vi "svx_Map Domains for Limit Testing.vi"(0 "X signal":dbl[](array[numeric]), 1 "domain mapping":T2(ring), 5 "Y signal":dbl[](array[numeric]), 7 "X limit":dbl[](array[numeric]), 9 "Y limit":dbl[](array[numeric]), 11 "error in (no error)":errorcluster, 12 "interpolated plot mapping":T1(ring)) -> (4 "X signal out":dbl[](array[numeric]), 6 "Y signal out":dbl[](array[numeric]), 8 "X limit out":dbl[](array[numeric]), 10 "Y limit out":dbl[](array[numeric]) format="%.2f", 15 "error out":errorcluster)   [LabVIEW 2017]
uses:
  <vilib>/Analysis/1siggen.llb/Ramp Pattern by Samples.vi
  <vilib>/Analysis/NI_AALBase.lvlib
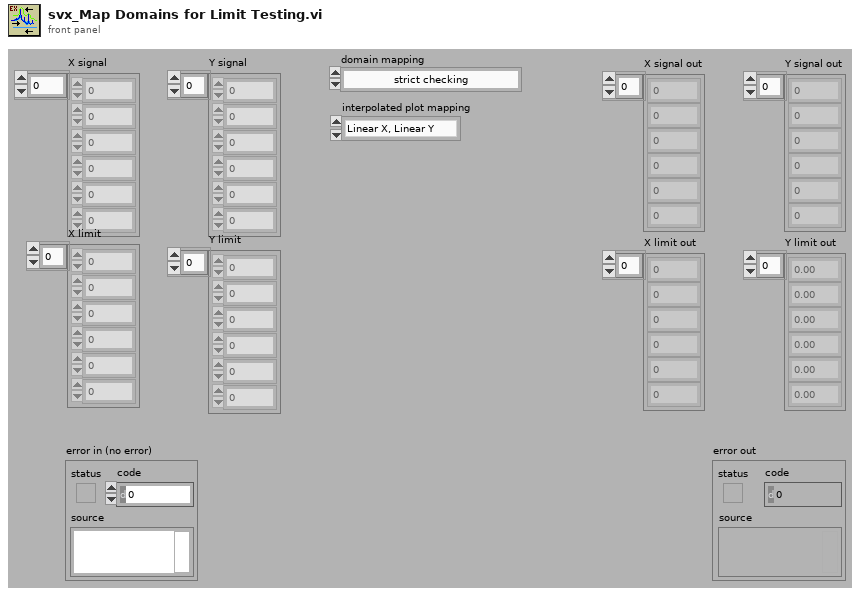
[diagram p1: front panel]
types:
  T1 = enum16{"Linear X, Linear Y", "Linear X, Log Y", "Log X, Linear Y", "Log X, Log Y"}
  T2 = enum16{"strict checking", "interpolate signal domain", "map limits to signal domain", "map signal to limit domain", "map signal and limits to unit domain"}
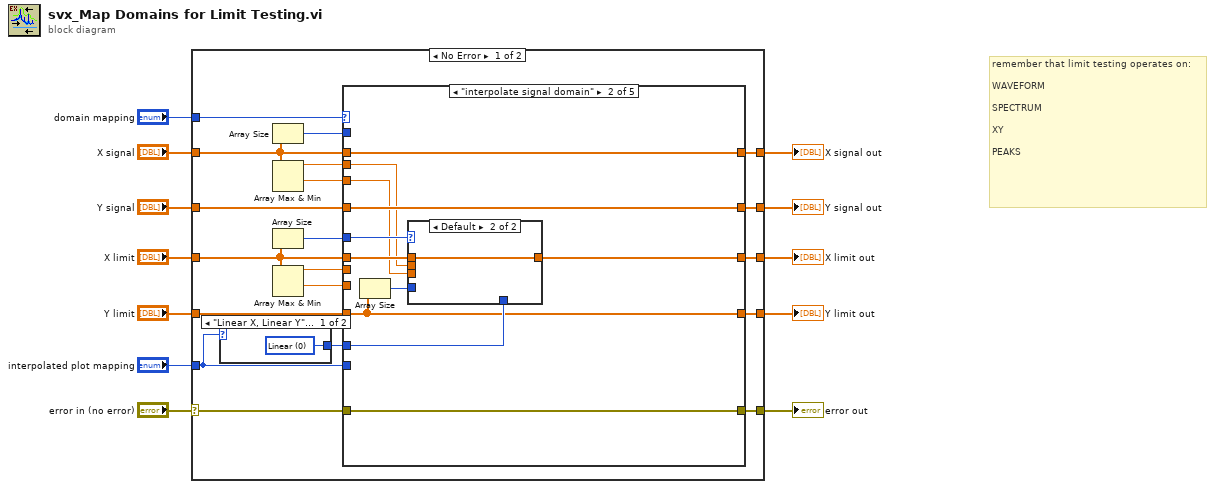
[diagram p0: block diagram]
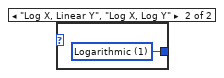
[diagram p2: hidden frame]
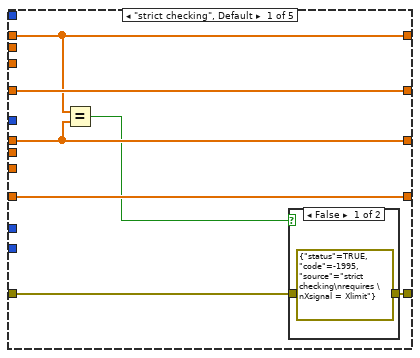
[diagram p3: hidden frame]
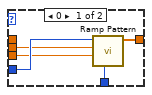
[diagram p5: hidden frame]
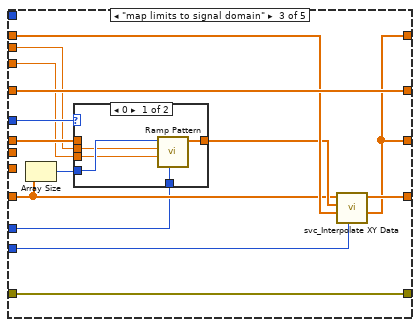
[diagram p6: hidden frame]
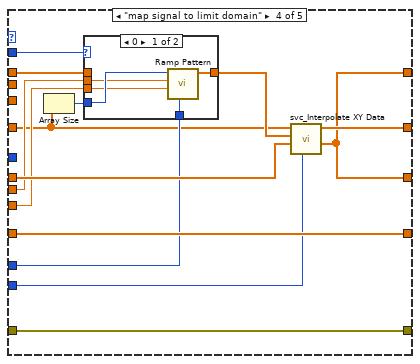
[diagram p8: hidden frame]
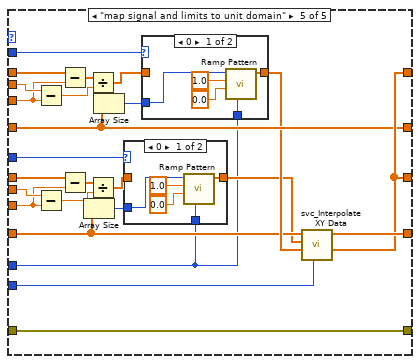
[diagram p10: hidden frame]
diagram:
  # "remember that limit testing operates on:\n\nWAVEFORM\n\nSPECTRUM\n\nXY\n\nPEAKS"
  n1 = case shown="No Error" "error in (no error)" {
    selector: "error in (no error)" -> [w24 w141]
    tunnel: "domain mapping" -> [w31 _]
    tunnel: "X signal" -> [w16 w140]
    tunnel: "X limit" -> [w18 w138]
    tunnel: [w30 w140] -> w9
    tunnel: "Y signal" -> [w29 w139]
    tunnel: [w28 w139] -> w7
    tunnel: [w27 w138] -> w6
    tunnel: "Y limit" -> [w26 w137]
    tunnel: [w25 w137] -> w4
    tunnel: [w23 w141] -> w2
    tunnel: "interpolated plot mapping" -> [w14 _]
    frame No Error {
      n2 = case shown="\"Linear X, Linear Y\", \"Linear X, Log Y\", Default" w14 {
        tunnel: [w32 w33] -> w13
        frame "Linear X, Linear Y", "Linear X, Log Y", Default {
          w32 = u16 0 items=["Linear", "Logarithmic"] ("type")
        }
        frame "Log X, Linear Y", "Log X, Log Y" {
          w33 = u16 1 items=["Linear", "Logarithmic"] ("type")
        }
      }
      n3 = Array Size(array=w16) -> (size(s)=w15:i32)
      n4 = Array Max & Min(array=w16) -> (max value=w20:dbl, min value=w19:dbl)  [unwired: 2 out]
      n5 = Array Size(array=w18) -> (size(s)=w17:i32)
      n6 = Array Max & Min(array=w18) -> (max value=w22:dbl, min value=w21:dbl)  [unwired: 2 out]
      n7 = case shown="\"interpolate signal domain\"" w31 {
        tunnel: w16 -> [w37 w45 w69 w84 w122]
        tunnel: w18 -> [w38 w50 w67 w87 w118]
        tunnel: [w37 w45 w60 w80 w113] -> w30
        tunnel: [w40 w52 w72 w91 w108] -> w28
        tunnel: w29 -> [w40 w52 w72 w81 w108]
        tunnel: [w38 w44 w60 w80 w113] -> w27
        tunnel: [w39 w43 w70 w92 w114] -> w25
        tunnel: w26 -> [w39 w43 w65 w92 w103]
        tunnel: w24 -> [w35 w53 w73 w93 w124]
        tunnel: [w34 w53 w73 w93 w124] -> w23
        tunnel: w22 -> [_ _ _ w86 w117]
        tunnel: w21 -> [_ _ _ w85 w116]
        tunnel: w20 -> [_ w48 w63 _ w123]
        tunnel: w19 -> [_ w47 w62 _ w120]
        tunnel: w14 -> [_ _ w71 w90 w112]
        tunnel: w17 -> [_ w51 w68 _ w104]
        tunnel: w15 -> [_ _ _ w88 w110]
        tunnel: w13 -> [_ w46 w61 w82 w100]
        frame "strict checking", Default {
          n8 = Equal?(x=w37, y=w38) -> (x = y?=w36:bool)
          n9 = case shown="False" w36 {
            tunnel: [errorcluster {"status"=TRUE, "code"=-1995, "source"="strict checking\nrequires \nXsignal = Xlimit"} ("error IO") w42] -> w34
            tunnel: w35 -> [_ w42]
            frame False {
            }
            frame True {
            }
          }
        }
        frame "interpolate signal domain" {
          n10 = Array Size(array=w43) -> (size(s)=w49:i32)
          n11 = case shown="Default" w51 {
            tunnel: w50 -> [_ w59]
            tunnel: [w57 w59] -> w44
            tunnel: w49 -> [w58 _]
            tunnel: w48 -> [w56 _]
            tunnel: w47 -> [w55 _]
            tunnel: w46 -> [w54 _]
            frame 0 {
              n12 = call-poly <vilib>:"Ramp Pattern.vi"("type"=w54, "start"=w55, "end"=w56, "samples"=w58) -> ("Ramp Pattern"=w57:dbl[])  [unwired: 6 in, 1 out]
            }
            frame Default {
            }
          }
        }
        frame "map limits to signal domain" {
          n13 = Array Size(array=w65) -> (size(s)=w64:i32)
          n14 = case shown="0" w68 {
            tunnel: w67 -> [_ w79]
            tunnel: [w77 w79] -> w66
            tunnel: w64 -> [w78 _]
            tunnel: w63 -> [w76 _]
            tunnel: w62 -> [w75 _]
            tunnel: w61 -> [w74 _]
            frame 0 {
              n15 = call-poly <vilib>:"Ramp Pattern.vi"("type"=w74, "start"=w75, "end"=w76, "samples"=w78) -> ("Ramp Pattern"=w77:dbl[])  [unwired: 6 in, 1 out]
            }
            frame Default {
            }
          }
          n16 = call <vilib>:"svc_Interpolate XY Data.vi"("interpolated plot mapping"=w71, "test X"=w69, "limit X"=w66, "limit Y"=w65) -> ("xi used"=w60:dbl[], "yi"=w70:dbl[])  [unwired: 6 in]
        }
        frame "map signal to limit domain" {
          n17 = Array Size(array=w81) -> (size(s)=w89:i32)
          n18 = case shown="0" w88 {
            tunnel: w84 -> [_ w99]
            tunnel: [w97 w99] -> w83
            tunnel: w89 -> [w98 _]
            tunnel: w86 -> [w96 _]
            tunnel: w85 -> [w95 _]
            tunnel: w82 -> [w94 _]
            frame 0 {
              n19 = call-poly <vilib>:"Ramp Pattern.vi"("type"=w94, "start"=w95, "end"=w96, "samples"=w98) -> ("Ramp Pattern"=w97:dbl[])  [unwired: 6 in, 1 out]
            }
            frame Default {
            }
          }
          n20 = call <vilib>:"svc_Interpolate XY Data.vi"("interpolated plot mapping"=w90, "test X"=w87, "limit X"=w83, "limit Y"=w81) -> ("xi used"=w80:dbl[], "yi"=w91:dbl[])  [unwired: 6 in]
        }
        frame "map signal and limits to unit domain" {
          n21 = Subtract(x=w123, y=w120) -> (x-y=w109:dbl)
          n22 = Subtract(x=w117, y=w116) -> (x-y=w115:dbl)
          n23 = Subtract(x=w122, y=w120) -> (x-y=w121:dbl[])
          n24 = Subtract(x=w118, y=w116) -> (x-y=w119:dbl[])
          n25 = Array Size(array=w103) -> (size(s)=w105:i32)
          n26 = Divide(x=w121, y=w109) -> (x/y=w107:dbl[])
          n27 = Divide(x=w119, y=w115) -> (x/y=w102:dbl[])
          n28 = Array Size(array=w108) -> (size(s)=w111:i32)
          n29 = case shown="0" w104 {
            tunnel: w102 -> [_ w130]
            tunnel: [w125 w130] -> w101
            tunnel: w105 -> [w129 _]
            tunnel: w100 -> [w128 _]
            frame 0 {
              n30 = call-poly <vilib>:"Ramp Pattern.vi"("type"=w128, "start"=0.0, "end"=1.0, "samples"=w129) -> ("Ramp Pattern"=w125:dbl[])  [unwired: 6 in, 1 out]
            }
            frame Default {
            }
          }
          n31 = case shown="0" w110 {
            tunnel: w107 -> [_ w136]
            tunnel: [w134 w136] -> w106
            tunnel: w111 -> [w135 _]
            tunnel: w100 -> [w133 _]
            frame 0 {
              n32 = call-poly <vilib>:"Ramp Pattern.vi"("type"=w133, "start"=0.0, "end"=1.0, "samples"=w135) -> ("Ramp Pattern"=w134:dbl[])  [unwired: 6 in, 1 out]
            }
            frame Default {
            }
          }
          n33 = call <vilib>:"svc_Interpolate XY Data.vi"("interpolated plot mapping"=w112, "test X"=w106, "limit X"=w101, "limit Y"=w103) -> ("xi used"=w113:dbl[], "yi"=w114:dbl[])  [unwired: 6 in]
        }
      }
    }
    frame Error {
    }
  }
  "X signal out" <- w9
  "Y signal out" <- w7
  "X limit out" <- w6
  "Y limit out" <- w4
  "error out" <- w2
